vi "CreateCommands.vi"   [LabVIEW 2014]
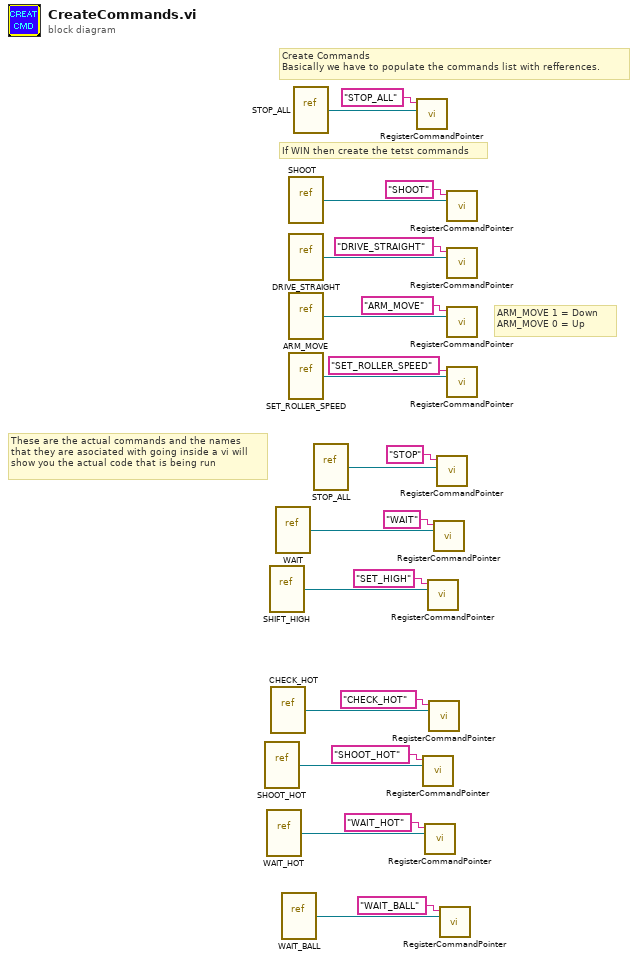
[diagram p0: block diagram]
diagram:
  # "These are the actual commands and the names \nthat they are asociated with going inside a vi will\nshow you the actual code that is being run"
  # "ARM_MOVE 1 = Down\nARM_MOVE 0 = Up"
  # "If WIN then create the tetst commands"
  # "Create Commands\nBasically we have to populate the commands list with refferences."
  n1 = vi-ref "SHOOT_HOT.vi"() -> (w9:refnum<vi>)
  n2 = vi-ref "WAIT_HOT.vi"() -> (w4:refnum<vi>)
  n3 = vi-ref "SHIFT_HIGH.vi"() -> (w8:refnum<vi>)
  n4 = vi-ref "CHECK_HOT.vi"() -> (w11:refnum<vi>)
  n5 = vi-ref "WAIT.vi"() -> (w13:refnum<vi>)
  n6 = vi-ref "WAIT_BALL.vi"() -> (w1:refnum<vi>)
  n7 = vi-ref "SHOOT.vi"() -> (w21:refnum<vi>)
  n8 = vi-ref "DRIVE_STRAIGHT.vi"() -> (w19:refnum<vi>)
  n9 = vi-ref "ARM_MOVE.vi"() -> (w17:refnum<vi>)
  n10 = vi-ref "SET_ROLLER_SPEED.vi"() -> (w15:refnum<vi>)
  n11 = vi-ref "STOP_ALL.vi"() -> (w23:refnum<vi>)
  n12 = vi-ref "STOP_ALL.vi"() -> (w6:refnum<vi>)
  n13 = call "RegisterCommandPointer.vi"("Strict-Typed VI Refnum"=w23, "Name"="STOP_ALL") -> ()  [unwired: 10 in]
  n14 = call "RegisterCommandPointer.vi"("Strict-Typed VI Refnum"=w9, "Name"="SHOOT_HOT") -> ()  [unwired: 10 in]
  n15 = call "RegisterCommandPointer.vi"("Strict-Typed VI Refnum"=w4, "Name"="WAIT_HOT") -> ()  [unwired: 10 in]
  n16 = call "RegisterCommandPointer.vi"("Strict-Typed VI Refnum"=w8, "Name"="SET_HIGH") -> ()  [unwired: 10 in]
  n17 = call "RegisterCommandPointer.vi"("Strict-Typed VI Refnum"=w11, "Name"="CHECK_HOT") -> ()  [unwired: 10 in]
  n18 = call "RegisterCommandPointer.vi"("Strict-Typed VI Refnum"=w13, "Name"="WAIT") -> ()  [unwired: 10 in]
  n19 = call "RegisterCommandPointer.vi"("Strict-Typed VI Refnum"=w6, "Name"="STOP") -> ()  [unwired: 10 in]
  n20 = call "RegisterCommandPointer.vi"("Strict-Typed VI Refnum"=w1, "Name"="WAIT_BALL") -> ()  [unwired: 10 in]
  n21 = call "RegisterCommandPointer.vi"("Strict-Typed VI Refnum"=w21, "Name"="SHOOT") -> ()  [unwired: 10 in]
  n22 = call "RegisterCommandPointer.vi"("Strict-Typed VI Refnum"=w19, "Name"="DRIVE_STRAIGHT") -> ()  [unwired: 10 in]
  n23 = call "RegisterCommandPointer.vi"("Strict-Typed VI Refnum"=w17, "Name"="ARM_MOVE") -> ()  [unwired: 10 in]
  n24 = call "RegisterCommandPointer.vi"("Strict-Typed VI Refnum"=w15, "Name"="SET_ROLLER_SPEED") -> ()  [unwired: 10 in]
